vi "JoystickLog.vi"(6 "Axes":T1, 7 "PID y":T2={"proportional gain (Kc)"=0.7000000000000001, "integral time (Ti, min)"=0.0, "derivative time (Td, min)"=0.0} {"derivative time (Td, min)" format="%.3f"; "integral time (Ti, min)" format="%.3f"; "proportional gain (Kc)" format="%.3f"}, 9 "XMAXMIN":cluster{"output high":dbl, "output low":dbl}, 10 "YMAXMIN":cluster{"output high":dbl, "output low":dbl}, 11 "PID x":T2={"proportional gain (Kc)"=0.7000000000000001, "integral time (Ti, min)"=0.0, "derivative time (Td, min)"=0.0} {"derivative time (Td, min)" format="%.3f"; "integral time (Ti, min)" format="%.3f"; "proportional gain (Kc)" format="%.3f"}) -> (2 "upper limit":dbl, 3 "upper limit 2":dbl)   [LabVIEW 2013]
uses:
  Robot Global Data.vi
  <vilib>/addons/control/pid/pid.llb/PID (DBL).vi
  <vilib>/addons/control/pid/NI_PID_pid.lvlib
panel:
  in  "CubicY":bool
  in  "CubicX":bool
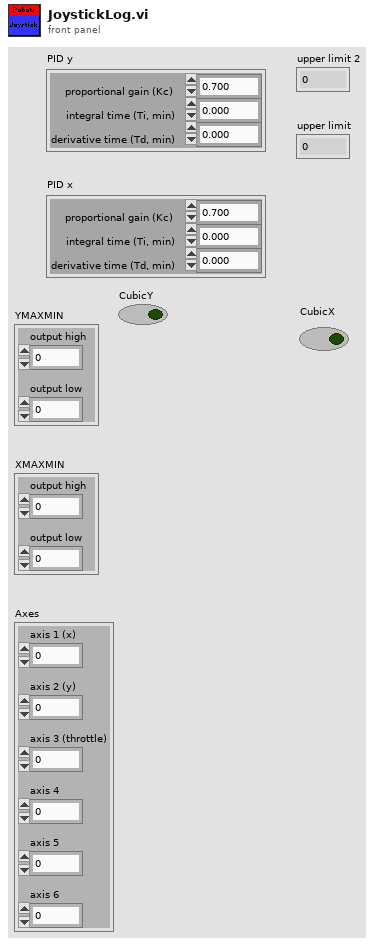
[diagram p1: front panel]
types:
  T1 = cluster{"axis 1 (x)":dbl, "axis 2 (y)":dbl, "axis 3 (throttle)":dbl, "axis 4":dbl, "axis 5":dbl, "axis 6":dbl}
  T2 = cluster{"proportional gain (Kc)":dbl, "integral time (Ti, min)":dbl, "derivative time (Td, min)":dbl}
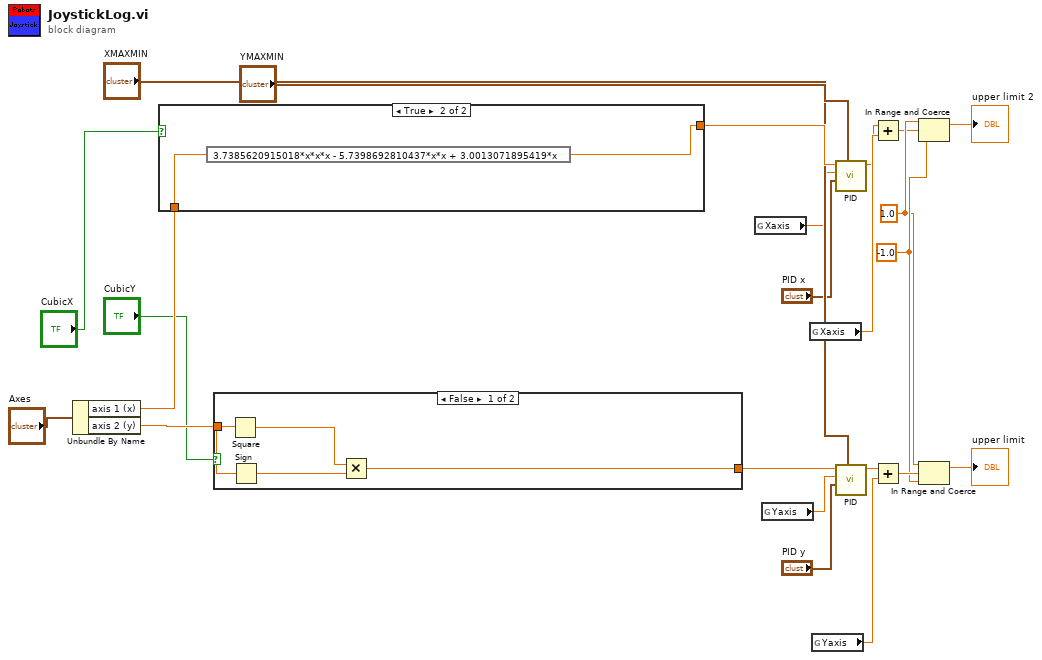
[diagram p0: block diagram]
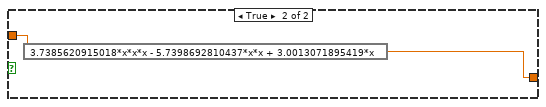
[diagram p2: hidden frame]
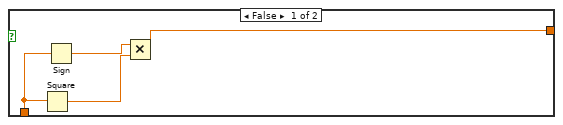
[diagram p3: hidden frame]
diagram:
  w16 = -1.0 ("upper limit")
  w15 = 1.0 ("upper limit")
  n1 = Unbundle By Name("Axes") -> ("axis 1 (x)"=w21:dbl, "axis 2 (y)"=w20:dbl)
  n2 = case shown="True" "CubicX" {
    tunnel: w21 -> [w27 w29]
    tunnel: [w25 w28] -> w18
    frame False {
      n3 = Square(x=w27) -> (x^2=w24:dbl)
      n4 = Sign(1:w27) -> (0:w26:dbl)
      n5 = Multiply(x=w26, y=w24) -> (x*y=w25:dbl)
    }
    frame True {
      n6 = expression code="3.7385620915018*x*x*x - 5.7398692810437*x*x + 3.0013071895419*x"(w29) -> (w28:dbl)
    }
  }
  n7 = case shown="False" "CubicY" {
    tunnel: w20 -> [w33 w34]
    tunnel: [w31 w35] -> w19
    frame False {
      n8 = Square(x=w33) -> (x^2=w30:dbl)
      n9 = Sign(1:w33) -> (0:w32:dbl)
      n10 = Multiply(x=w30, y=w32) -> (x*y=w31:dbl)
    }
    frame True {
      n11 = expression code="3.7385620915018*x*x*x - 5.7398692810437*x*x + 3.0013071895419*x"(w34) -> (w35:dbl)
    }
  }
  n12 = global read "Robot Global Data.vi" "Xaxis"() -> (w8:dbl)
  n13 = global read "Robot Global Data.vi" "Yaxis"() -> (w9:dbl)
  n14 = global read "Robot Global Data.vi" "Xaxis"() -> (w12:dbl)
  n15 = global read "Robot Global Data.vi" "Yaxis"() -> (w13:dbl)
  n16 = call-poly <vilib>:"PID.vi"("output range"="YMAXMIN", "PID gains"="PID x", "process variable"=w8, "setpoint"=w18) -> ("output"=w7:dbl)  [unwired: 6 in, 1 out]
  n17 = call-poly <vilib>:"PID.vi"("output range"="XMAXMIN", "PID gains"="PID y", "process variable"=w9, "setpoint"=w19) -> ("output"=w6:dbl)  [unwired: 6 in, 1 out]
  n18 = Add(x=w7, y=w12) -> (x+y=w14:dbl)
  n19 = Add(x=w6, y=w13) -> (x+y=w17:dbl)
  n20 = In Range and Coerce(upper limit=w15, x=w14, lower limit=w16) -> (coerced(x)=→"upper limit 2":dbl)  [unwired: 1 out]
  n21 = In Range and Coerce(upper limit=w15, x=w17, lower limit=w16) -> (coerced(x)=→"upper limit":dbl)  [unwired: 1 out]
